vi "B-Lockin_time.vi"(8 "stop":bool, 9 "IPS VISA resource name":refnum<visa-resource-name>="GPIB0::24::INSTR", 10 "Comments":string="SA03036H.20180409\ncool down\nI+/I-: 2/3 200uV ac+ 250udc offset, 13Hz\nV1+/V1-: 8/4\nV2+/V2-: 6/28\nV3+/V3-: 27/7\n", 11 "folder name":string="cooldown") -> (1 "X1":cluster{"Y":dbl[], "Y":dbl[]}[](graph), 3 "Temp vs Time":cluster{"Y":dbl[], "Y":dbl[]}[](graph), 5 "X4":cluster{"Y":dbl[], "Y":dbl[]}[](graph))   [LabVIEW 2016, in "Transport.lvclass"]
uses:
  Transport.lvclass
  subVI/ITX_Global.vi
  <userlib>/LevyLab/LV to ITX/LVtoITX.lvclass
panel:
  in  "Tab Control":T1(tab)
  in  "milliseconds to wait":u32=1000
  in  "Lockins":i32[](array[numeric])=[0, 1, 2, 3, 4, 5, 6, 7]
  out "Array X":dbl[](array[numeric])
  out "Array Y":dbl[](array[numeric])
  in  "append to file? (new file:F)":bool
  out "X0":cluster{"Y":dbl[], "Y":dbl[]}[](graph)
  out "X2":cluster{"Y":dbl[], "Y":dbl[]}[](graph)
  out "X3":cluster{"Y":dbl[], "Y":dbl[]}[](graph)
  out "X5":cluster{"Y":dbl[], "Y":dbl[]}[](graph)
  out "R vs time":cluster{"Y":dbl[], "Y":dbl[]}[](graph)
  in  "V1":i32
  in  "Current 1":i32
  out "B vs Time":cluster{"Y":dbl[], "Y":dbl[]}[](graph)
  out "R vs T":cluster{"Y":dbl[], "Y":dbl[]}[](graph)
  # "0,1,2,3 ect."
  # "NOT READING MAGNETIC FIELD -- 6/16/2017, Patrick"
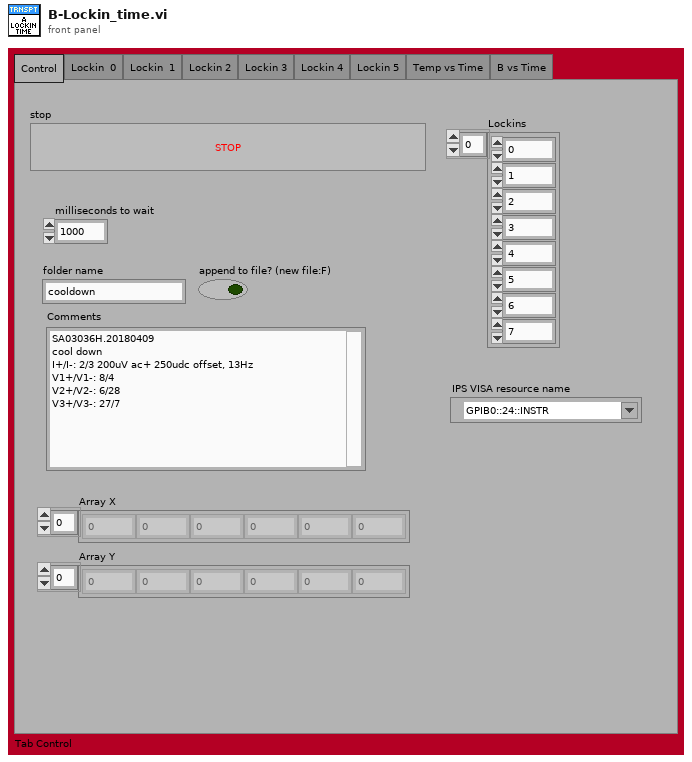
[diagram p1: front panel]
types:
  T1 = enum32{"Control", "Lockin  0", "Lockin  1", "Lockin 2", "Lockin 3", "Lockin 4", "Lockin 5", "Temp vs Time", "B vs Time"}
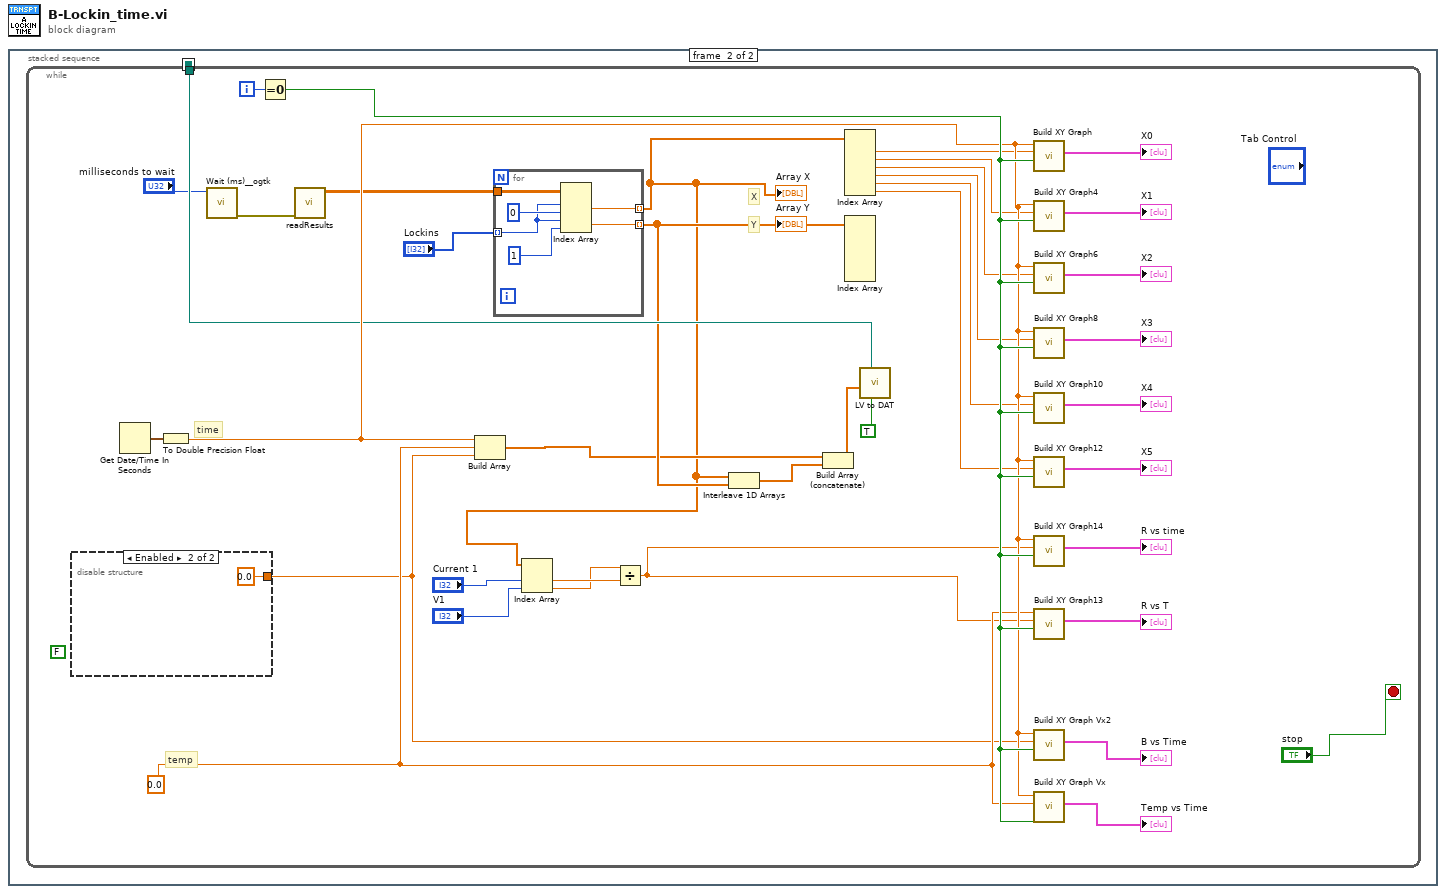
[diagram p0: block diagram]
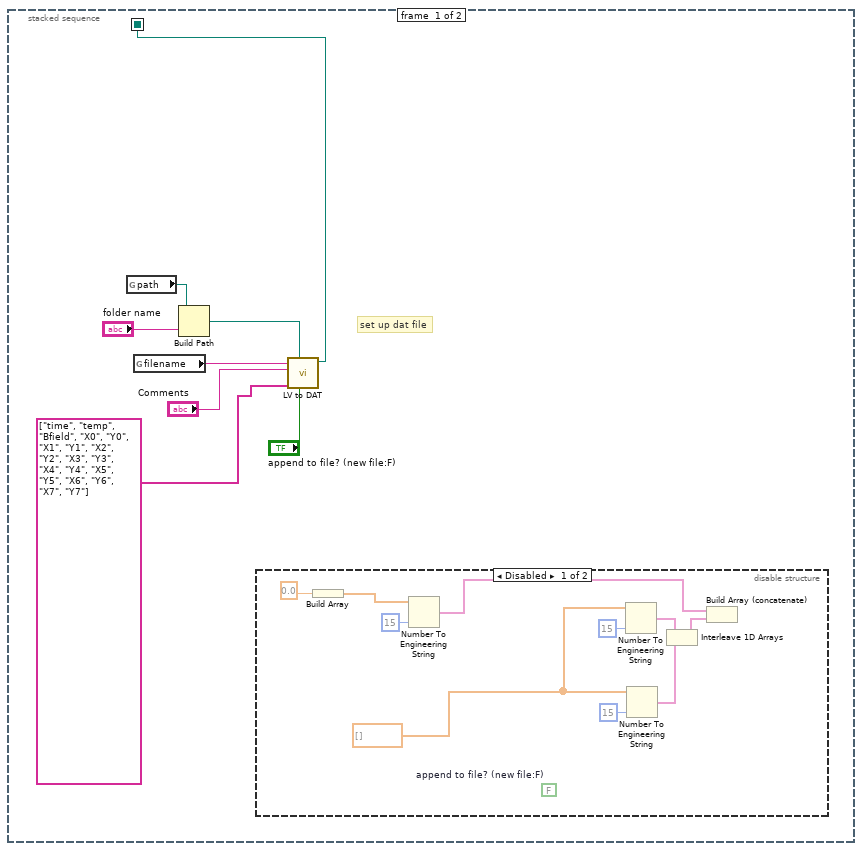
[diagram p2: hidden frame]
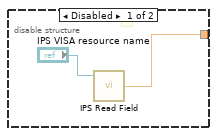
[diagram p4: hidden frame]
diagram:
  n1 = stacked-sequence {
    seq-local: [w3 _] -> [_ w19]
    frame #0 {
      # "set up dat file"
      n2 = global read "ITX_Global.vi" "path"() -> (w8:path)
      n3 = global read "ITX_Global.vi" "filename"() -> (w4:string)
      n4 = Build Path(base path=w8, name or relative path="folder name") -> (appended path=w1:path)
      n5 = disable-structure shown="Disabled" {
        frame Disabled {
          w9 = dbl[] []
          (unwired) FALSE  # append to file? (new file:F)
          n6 = Build Array(0.0) -> (w15:dbl[])
          n7 = Number To Engineering String(2:i16 15 ("precision (6)"), 4:w15) -> (0:w14:string[])  [unwired: 2 out]
          n8 = Number To Engineering String(2:i16 15 ("precision (6)"), 4:w9) -> (0:w13:string[])  [unwired: 2 out]
          n9 = Number To Engineering String(2:i16 15 ("precision (6)"), 4:w9) -> (0:w12:string[])  [unwired: 2 out]
          n10 = Interleave 1D Arrays(w13, w12) -> (w11:string[])
          n11 = Build Array (concatenate)(w14, w11) -> ()  [unwired: 1 out]
        }
        frame Enabled {
        }
      }
      n12 = call <userlib>:"LV to DAT.vi"("append to file? (new file:F)"="append to file? (new file:F)", "path"=w1, "wavenames (.Vx, etc)"=string[] ["time", "temp", "Bfield", "X0", "Y0", "X1", "Y1", "X2", "Y2", "X3", "Y3", "X4", "Y4", "X5", "Y5", "X6", "Y6", "X7", "Y7"], "Comments"="Comments", "filename"=w4) -> ("new file path"=w3:path)  [unwired: 6 in]
    }
    frame #1 {
      n13 = while {
        tunnel: w19 -> [w53]
        i -> [w58]
        stop <- "stop" stop-if-true
        (unwired) FALSE ("Boolean")
        w55 = 0.0 ("Temp")
        # "Y"
        # "X"
        # "time"
        # "temp"
        n14 = disable-structure shown="Enabled" {
          disable-tunnel: [w66 0.0 ("Field (T)")] -> w54
          frame Disabled {
            # "B"
            n15 = call "IPS Read Field.vi"("VISA resource name (COM Port of Prologix Device)"="IPS VISA resource name") -> ("Field (T)"=w66:dbl)  [unwired: 2 in, 2 out]
          }
          frame Enabled {
          }
        }
        n16 = Get Date/Time In Seconds() -> (seconds since 1Jan1904=w50:timestamp)
        n17 = To Double Precision Float(number=w50) -> (double precision float=w56:dbl)
        n18 = call <userlib>:"Wait (ms)__ogtk.vi"("milliseconds to wait"="milliseconds to wait") -> ("error out"=w48:errorcluster)  [unwired: 9 in, 1 out]
        n19 = Equal To 0?(x=w58) -> (x = 0?=w57:bool)
        n20 = call <userlib>:"readResults.vi"("error in (no error)"=w48) -> ("Results"=w51:dbl[][])  [unwired: 9 in, 1 out]
        n21 = Build Array(w56, w55, w54) -> (w21:dbl[])
        n22 = for {
          tunnel: w51 -> [w61]
          tunnel: "Lockins" -> [w62] mode=indexing
          tunnel: [w59] -> w20 mode=indexing
          tunnel: [w60] -> w24 mode=indexing
          n23 = Index Array(array=w61, index (row) #1=w62, index (col) #1=0 ("disabled index (col)"), index (row) #2=w62, index (col) #2=1 ("disabled index (col)")) -> (element #1=w59:dbl, element #2=w60:dbl)
        }
        "Array X" <- w20
        "Array Y" <- w24
        n24 = Index Array(array=w20, index #1="Current 1", index #2="V1") -> (element #1=w30:dbl, element #2=w25:dbl)
        n25 = Divide(x=w25, y=w30) -> (x/y=w27:dbl)
        n26 = Interleave 1D Arrays(w20, w24) -> (w26:dbl[])
        n27 = Build Array (concatenate)(w21, w26) -> (w23:dbl[])
        n28 = Index Array(array=w20) -> (element #1=w45:dbl, element #2=w43:dbl, element #3=w41:dbl, element #4=w39:dbl, element #5=w37:dbl, element #6=w35:dbl)  [unwired: 6 in]
        n29 = Index Array(array=w24) -> ()  [unwired: 6 in, 6 out]
        n30 = call <userlib>:"LV to DAT.vi"("append to file? (new file:F)"=TRUE, "path"=w53, "Data"=w23) -> ()  [unwired: 8 in, 1 out]
        n31 = call "Build XY Graph"("Reset"=w57, "Y Input"=w45, "X Input"=w56) -> ("XY Graph"=→"X0":cluster{"Y":dbl[], "Y":dbl[]}[])  [unwired: 2 in, 6 out]
        n32 = call "Build XY Graph4"("Reset"=w57, "Y Input"=w43, "X Input"=w56) -> ("XY Graph"=→"X1":cluster{"Y":dbl[], "Y":dbl[]}[])  [unwired: 2 in, 6 out]
        n33 = call "Build XY Graph6"("Reset"=w57, "Y Input"=w41, "X Input"=w56) -> ("XY Graph"=→"X2":cluster{"Y":dbl[], "Y":dbl[]}[])  [unwired: 2 in, 6 out]
        n34 = call "Build XY Graph8"("Reset"=w57, "Y Input"=w39, "X Input"=w56) -> ("XY Graph"=→"X3":cluster{"Y":dbl[], "Y":dbl[]}[])  [unwired: 2 in, 6 out]
        n35 = call "Build XY Graph10"("Reset"=w57, "Y Input"=w37, "X Input"=w56) -> ("XY Graph"=→"X4":cluster{"Y":dbl[], "Y":dbl[]}[])  [unwired: 2 in, 6 out]
        n36 = call "Build XY Graph12"("Reset"=w57, "Y Input"=w35, "X Input"=w56) -> ("XY Graph"=→"X5":cluster{"Y":dbl[], "Y":dbl[]}[])  [unwired: 2 in, 6 out]
        n37 = call "Build XY Graph14"("Reset"=w57, "Y Input"=w27, "X Input"=w56) -> ("XY Graph"=→"R vs time":cluster{"Y":dbl[], "Y":dbl[]}[])  [unwired: 2 in, 6 out]
        n38 = call "Build XY Graph13"("Reset"=w57, "Y Input"=w27, "X Input"=w55) -> ("XY Graph"=→"R vs T":cluster{"Y":dbl[], "Y":dbl[]}[])  [unwired: 2 in, 6 out]
        n39 = call "Build XY Graph Vx2"("Reset"=w57, "Y Input"=w54, "X Input"=w56) -> ("XY Graph"=→"B vs Time":cluster{"Y":dbl[], "Y":dbl[]}[])  [unwired: 2 in, 6 out]
        n40 = call "Build XY Graph Vx"("Reset"=w57, "Y Input"=w55, "X Input"=w56) -> ("XY Graph"=→"Temp vs Time":cluster{"Y":dbl[], "Y":dbl[]}[])  [unwired: 2 in, 6 out]
      }
    }
  }
